vi "Store_Missed_Events.vi"(7 "initTime":u32, 9 "variables":string, 10 "expId":string, 11 "LabVIEW Web Service Request":refnum<class "Web Request.lvclass">) -> (2 "path":path, 3 "LabVIEW Web Service Request out":refnum<class "Web Request.lvclass">)   [LabVIEW 2014]
doc: "Waits for the client to reconnect and stores all missed events"
uses:
  Configuration/Global_Configurations.vi
  <vilib>/wsapi/Web Request.lvclass
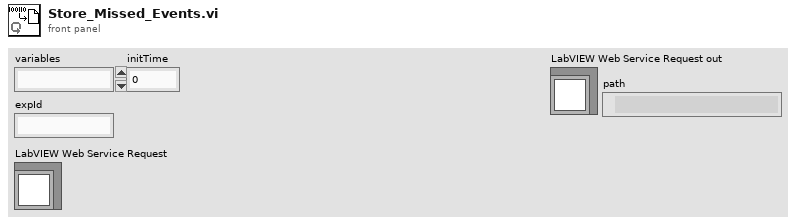
[diagram p1: front panel]
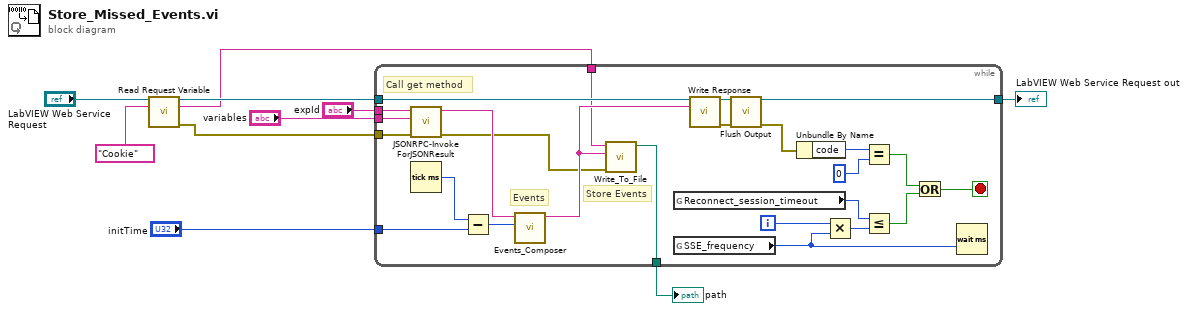
[diagram p0: block diagram]
diagram:
  n1 = call <vilib>:"Read Request Variable.vi"("LabVIEW Web Service Request"="LabVIEW Web Service Request", "variable name"="Cookie") -> ("LabVIEW Web Service Request out"=w3:refnum<class "Web Request.lvclass">, "value"=w1:string, "error out"=w2:errorcluster)  [unwired: 11 in]
  n2 = while {
    tunnel: w3 -> [w13]
    tunnel: "expId" -> [w31]
    tunnel: "initTime" -> [w28]
    tunnel: [w27] -> w7
    tunnel: "variables" -> [w25]
    tunnel: w2 -> [w15]
    tunnel: [w14] -> w6
    tunnel: w1 -> [w11]
    i -> [w22]
    stop <- w17 stop-if-true
    # "Store Events"
    # "Events"
    # "Call get method"
    n3 = call "JSONRPC-InvokeForJSONResult.vi"("error in"=w15, "variables"=w25, "expid"=w31) -> ("error out"=w12:errorcluster, "response"=w30:string)  [unwired: 7 in]
    n4 = Tick Count (ms)() -> (millisecond timer value=w29:u32)
    n5 = Subtract(x=w29, y=w28) -> (x-y=w24:u32)
    n6 = call "Events_Composer.vi"("time"=w24, "responsein"=w30) -> ("responseout"=w16:string)  [unwired: 9 in]
    n7 = call "Write_To_File.vi"("error in"=w12, "data"=w16, "cookie"=w11) -> ("path"=w14:path)  [unwired: 7 in, 1 out]
    n8 = global read "Global_Configurations.vi" "Reconnect_session_timeout"() -> (w20:u32)
    n9 = global read "Global_Configurations.vi" "SSE_frequency"() -> (w21:u32)
    n10 = call <vilib>:"Write Response.vi"("LabVIEW Web Service Request"=w13, "response string"=w16) -> ("LabVIEW Web Service Request out"=w34:refnum<class "Web Request.lvclass">, "error out"=w35:errorcluster)  [unwired: 12 in]
    n11 = call <vilib>:"Flush Output.vi"("LabVIEW Web Service Request"=w34, "error in (no error)"=w35) -> ("LabVIEW Web Service Request out"=w27:refnum<class "Web Request.lvclass">, "error out"=w26:errorcluster)  [unwired: 12 in]
    n12 = Unbundle By Name(w26) -> ("code"=w33:i32)
    n13 = Multiply(x=w22, y=w21) -> (x*y=w23:u32)
    n14 = Equal?(x=w33, y=0) -> (x = y?=w19:bool)
    n15 = Less Or Equal?(x=w20, y=w23) -> (x <= y?=w18:bool)
    n16 = Or(x=w19, y=w18) -> (x .or. y?=w17:bool)
    n17 = Wait (ms)(milliseconds to wait=w21) -> ()  [unwired: 1 out]
  }
  "LabVIEW Web Service Request out" <- w7
  "path" <- w6
